vi "FillMsgArray.vi"(1 "Input VOC msg Array":T1(array[cluster])) -> (0 "Clear msg Array":T1(array[cluster]))   [LabVIEW 2010]
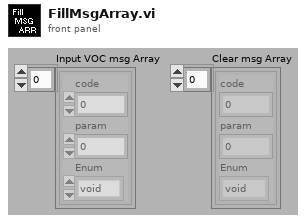
[diagram p1: front panel]
types:
  T1 = cluster{"code":i32, "param":i32, "Enum":enum16{"void", "byte", "int", "float"}}[]
  T2 = cluster{"code":i32, "param":i32, "Enum":enum32{"void", "byte", "int", "float"}}
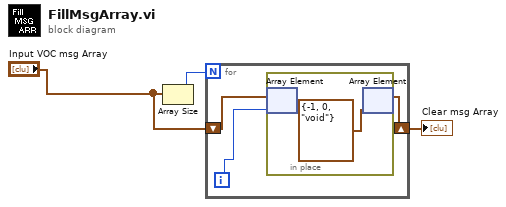
[diagram p0: block diagram]
diagram:
  n1 = Array Size(array="Input VOC msg Array") -> (size(s)=w3:i32)
  n2 = for {
    N: w3 -> [_]
    shift-right: [w4] -> w1
    shift-left: "Input VOC msg Array" -> [w6]
    i -> [w5]
    n3 = in-place {
      n4 = in-place-array #1(w6, w5) -> ()  [unwired: 1 out]
      n5 = in-place-array #1(T2 {"code"=-1, "param"=0, "Enum"=enum."void"} ("Cluster")) -> (w4:T1)  [unwired: 1 out]
    }
  }
  "Clear msg Array" <- w1
